vi "S2C_ExeScriptUpdateTest.vi"(8 "Error In":errorcluster, 10 "LastMeas?":bool, 11 "Status":T1) -> (0 "Error Out":errorcluster)   [LabVIEW 2015]
doc: "Determines the result for the currently executing line item, and updates the measurement and result in the data array."
uses:
  Controls/S2C_ResultStatus.ctl
  LVIS/Sub VIs/Globals/LVIS_IsGlobal.vi
  Globals/S2C_Globals.vi
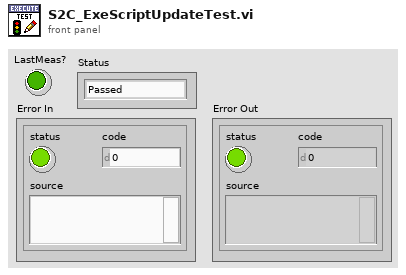
[diagram p1: front panel]
types:
  T1 = typedef "S2C_ResultStatus.ctl" = enum16{"Passed", "Failed", "Logged", "Aborted", "Error", "Testing...", "Paused", "No Record"}
  T2 = cluster{"EventStatus":string, "TestStatus":string, "MeasStatus":string}
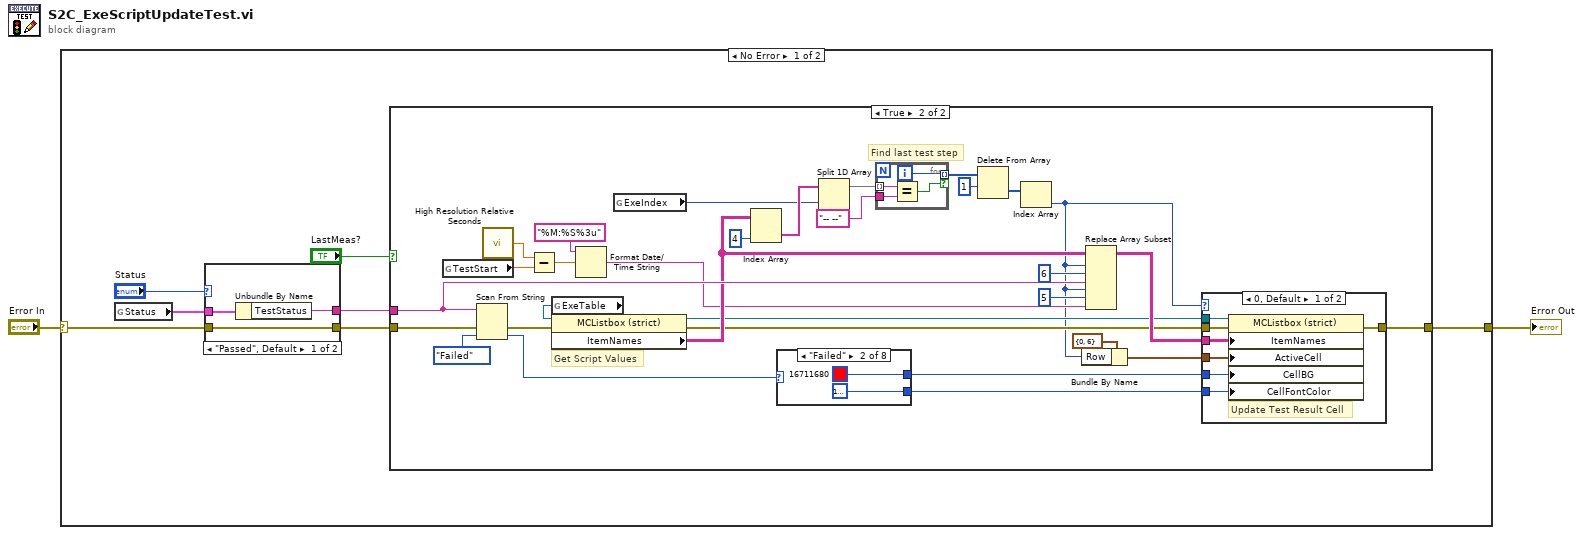
[diagram p0: block diagram]
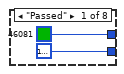
[diagram p4: hidden frame]
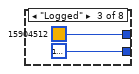
[diagram p5: hidden frame]
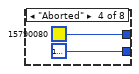
[diagram p6: hidden frame]
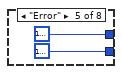
[diagram p7: hidden frame]
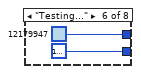
[diagram p8: hidden frame]
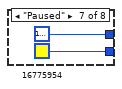
[diagram p9: hidden frame]
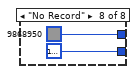
[diagram p10: hidden frame]
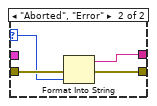
[diagram p11: hidden frame]
diagram:
  n1 = case shown="No Error" "Error In" {
    selector: "Error In" -> [w8 w77]
    tunnel: [w9 w77] -> w1
    frame No Error {
      n2 = global read "LVIS_IsGlobal.vi" "Status"() -> (w4:T2)
      n3 = case shown="\"Passed\", Default" "Status" {
        selector: "Status" -> [_ w75]
        tunnel: w8 -> [w72 w76]
        tunnel: [w72 w74] -> w6
        tunnel: [w70 w73] -> w5
        tunnel: w4 -> [w71 _]
        frame "Passed", Default {
          n4 = Unbundle By Name(w71) -> ("TestStatus"=w70:string)
        }
        frame "Aborted", "Error" {
          n5 = Format Into String(error in=w76, w75) -> (resulting string=w73:string, error out=w74:errorcluster)  [unwired: 2 in]
        }
      }
      n6 = case shown="True" "LastMeas?" {
        tunnel: [w10 w41] -> w9
        tunnel: w6 -> [w10 w40]
        tunnel: w5 -> [_ w39]
        frame False {
        }
        frame True {
          # "Find last test step"
          # "Get Script Values"
          n7 = global read "S2C_Globals.vi" "TestStart"() -> (w21:dbl)
          n8 = Scan From String(input string=w39, error in=w40, default 1=S2C_ResultStatus."Failed" ("y")) -> (error out=w28:errorcluster, output 1=w27:T1)  [unwired: 2 in, 2 out]
          n9 = call <vilib>:"High Resolution Relative Seconds.vi"() -> ("relative seconds"=w22:dbl)
          n10 = Subtract(x=w22, y=w21) -> (x-y=w20:dbl)
          n11 = global read "S2C_Globals.vi" "ExeTable"() -> (w29:refnum<vi>)
          n12 = property class="MCListbox (strict)"(reference=w29, error in=w28) -> (reference out=w24:refnum<vi>, error out=w26:errorcluster, "ItemNames"=w30:string[][])
          n13 = Format Date/Time String(time format string (%c)="%M:%S%3u", seconds (now)=w20) -> (date/time string=w17:string)  [unwired: 1 in]
          n14 = global read "S2C_Globals.vi" "ExeIndex"() -> (w36:i32)
          n15 = Index Array(array=w30, index (col)=4 ("disabled index (col)")) -> (element=w37:string[])  [unwired: 1 in]
          n16 = case shown="\"Failed\"" w27 {
            tunnel: [u32 46081 u32 16711680 u32 15904512 u32 15790080 u32 16777222 u32 12179947 u32 16777222 u32 9868950] -> w31
            tunnel: [u32 16777226 u32 16777226 u32 16777226 u32 16777222 u32 16777226 u32 16777222 u32 16775954 u32 16777226] -> w25
            frame "Passed" {
            }
            frame "Failed" {
            }
            frame "Logged" {
            }
            frame "Aborted" {
            }
            frame "Error" {
            }
            frame "Testing..." {
            }
            frame "Paused" {
            }
            frame "No Record" {
            }
          }
          n17 = Split 1D Array(array=w37, index=w36) -> (first subarray=w16:string[])  [unwired: 1 out]
          n18 = for {
            tunnel: w16 -> [w45] mode=indexing
            tunnel: "-- --" -> [w44]
            tunnel: [w43] -> w14 mode=indexing if=w42
            i -> [w43]
            n19 = Equal?(x=w45, y=w44) -> (x = y?=w42:bool)
          }
          n20 = Delete From Array(array=w14, length=1) -> (deleted portion=w12:i32[])  [unwired: 1 in, 1 out]
          n21 = Index Array(array=w12) -> (element=w11:i32)  [unwired: 1 in]
          n22 = Bundle By Name(cluster=cluster{"Row":i32, "Column":i32} {"Row"=0, "Column"=6} ("Active Cell:Active Cell"), "Row"=w11) -> (w32:cluster{"Row":i32, "Column":i32})
          n23 = Replace Array Subset(array=w30, new element #1=w39, index (row) #1=w11, index (col) #1=6 ("disabled index (col)"), new element #2=w17, index (row) #2=w11, index (col) #2=5 ("disabled index (col)")) -> (w34:string[][])
          n24 = case shown="0, Default" w11 {
            tunnel: w34 -> [w52 _]
            tunnel: w32 -> [w51 _]
            tunnel: w31 -> [w50 _]
            tunnel: [w49 w53] -> w41
            tunnel: w26 -> [w48 w53]
            tunnel: w25 -> [w47 _]
            tunnel: w24 -> [w46 _]
            frame 0, Default {
              # "Update Test Result Cell"
              n25 = property on="Property Node" class="MCListbox (strict)"(reference=w46, error in=w48, "ItemNames"=w52, "ActiveCell"=w51, "CellBG"=w50, "CellFontColor"=w47) -> (error out=w49:errorcluster)  [unwired: 1 out]
            }
            frame -1 {
            }
          }
        }
      }
    }
    frame Error {
    }
  }
  "Error Out" <- w1
